vi "SMO Activity Tree.vi"   [LabVIEW 2021, in "smo.lvlib" / "SMO.lvclass"]
uses:
  SMO.lvclass
  SMO.lvclass/SMO.ctl
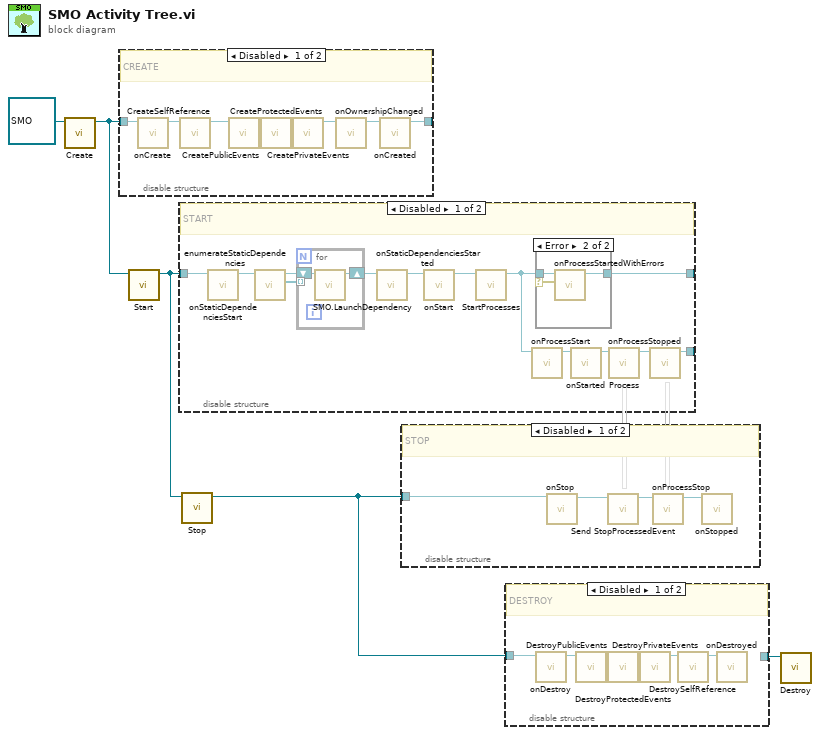
[diagram p0: block diagram]
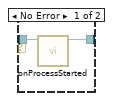
[diagram p4: hidden frame]
diagram:
  n1 = call "Create.vi"("SMO"=refnum<class "SMO.lvclass"> refnum) -> ("SMO out"=w3:refnum<class "SMO.lvclass">)  [unwired: 8 in, 2 out]
  n2 = disable-structure shown="Disabled" {
    disable-tunnel: w3 -> [w13 _]
    disable-tunnel: [w6 _] -> _
    frame Disabled {
      # "CREATE"
      n3 = call-dynamic "onCreate.vi"("SMO"=w13) -> ("SMO out"=w12:refnum<class "SMO.lvclass">)  [unwired: 9 in, 1 out]
      n4 = call-dynamic "CreateSelfReference.vi"("SMO"=w12) -> ("SMO out"=w11:refnum<class "SMO.lvclass">)  [unwired: 9 in, 1 out]
      n5 = call-dynamic "CreatePublicEvents.vi"("SMO"=w11) -> ("SMO out"=w10:refnum<class "SMO.lvclass">)  [unwired: 9 in, 1 out]
      n6 = call-dynamic "CreateProtectedEvents.vi"("SMO"=w10) -> ("SMO out"=w9:refnum<class "SMO.lvclass">)  [unwired: 9 in, 1 out]
      n7 = call-dynamic "CreatePrivateEvents.vi"("SMO"=w9) -> ("SMO out"=w8:refnum<class "SMO.lvclass">)  [unwired: 9 in, 1 out]
      n8 = call-dynamic "onOwnershipChanged.vi"("SMO in"=w8) -> ("SMO out"=w7:refnum<class "SMO.lvclass">)  [unwired: 9 in, 1 out]
      n9 = call-dynamic "onCreated.vi"("SMO"=w7) -> ("SMO out"=w6:refnum<class "SMO.lvclass">)  [unwired: 9 in, 1 out]
    }
    frame Enabled {
    }
  }
  n10 = call "Start.vi"("SMO"=w3) -> ("SMO out"=w4:refnum<class "SMO.lvclass">)  [unwired: 9 in, 1 out]
  n11 = disable-structure shown="Disabled" {
    disable-tunnel: w4 -> [w26 _]
    disable-tunnel: [w18 _] -> _
    disable-tunnel: [w17 _] -> _
    frame Disabled {
      # "START"
      n12 = call-dynamic "onStaticDependenciesStart.vi"("SMO"=w26) -> ("SMO out"=w24:refnum<class "SMO.lvclass">)  [unwired: 9 in, 1 out]
      n13 = call-dynamic "enumerateStaticDependencies.vi"("SMO"=w24) -> ("Static Dependencies"=w22:refnum<class "Dependency.lvclass">[], "SMO out"=w23:refnum<class "SMO.lvclass">)  [unwired: 8 in, 1 out]
      n14 = for {
        shift-right: [w33] -> w25
        shift-left: w23 -> [w32]
        tunnel: w22 -> [_] mode=indexing
        n15 = call "SMO.LaunchDependency.vi"("SMO in"=w32) -> ("SMO out"=w33:refnum<class "SMO.lvclass">)  [unwired: 7 in, 3 out]
      }
      n16 = call-dynamic "onStaticDependenciesStarted.vi"("SMO"=w25) -> ("SMO out"=w21:refnum<class "SMO.lvclass">)  [unwired: 9 in, 1 out]
      n17 = call-dynamic "onStart.vi"("SMO"=w21) -> ("SMO out"=w20:refnum<class "SMO.lvclass">)  [unwired: 9 in, 1 out]
      n18 = call "StartProcesses.vi"("SMO"=w20) -> ("SMO out"=w19:refnum<class "SMO.lvclass">)  [unwired: 9 in, 1 out]
      n19 = call-dynamic "onProcessStart.vi"("SMO"=w19) -> ("SMO out"=w16:refnum<class "SMO.lvclass">)  [unwired: 9 in, 1 out]
      n20 = case shown="Error" {
        selector: _ -> [_ w29]
        tunnel: w19 -> [w28 w31]
        tunnel: [w27 w30] -> w17
        frame No Error {
          n21 = call-dynamic "onProcessStarted.vi"("SMO"=w28) -> ("SMO out"=w27:refnum<class "SMO.lvclass">)  [unwired: 9 in, 1 out]
        }
        frame Error {
          n22 = call-dynamic "onProcessStartedWithErrors.vi"("Start error"=w29, "SMO"=w31) -> ("SMO out"=w30:refnum<class "SMO.lvclass">)  [unwired: 8 in, 1 out]
        }
      }
      n23 = call-dynamic "onStarted.vi"("SMO"=w16) -> ("SMO out"=w15:refnum<class "SMO.lvclass">)  [unwired: 9 in, 1 out]
      n24 = call-dynamic "Process.vi"("SMO"=w15) -> ("SMO out"=w14:refnum<class "SMO.lvclass">)  [unwired: 9 in, 1 out]
      n25 = call-dynamic "onProcessStopped.vi"("SMO"=w14) -> ("SMO out"=w18:refnum<class "SMO.lvclass">)  [unwired: 9 in, 1 out]
    }
    frame Enabled {
    }
  }
  n26 = call "Stop.vi"("SMO"=w4) -> ("SMO out"=w2:refnum<class "SMO.lvclass">)  [unwired: 9 in, 1 out]
  n27 = disable-structure shown="Disabled" {
    disable-tunnel: w2 -> [w37 _]
    frame Disabled {
      # "STOP"
      n28 = call-dynamic "onStop.vi"("SMO"=w37) -> ("SMO out"=w34:refnum<class "SMO.lvclass">)  [unwired: 9 in, 1 out]
      n29 = call "Send StopProcessedEvent.vi"("SMO"=w34) -> ("SMO out"=w35:refnum<class "SMO.lvclass">)  [unwired: 9 in, 1 out]
      n30 = call-dynamic "onProcessStop.vi"("SMO"=w35) -> ("SMO out"=w36:refnum<class "SMO.lvclass">)  [unwired: 9 in, 1 out]
      n31 = call-dynamic "onStopped.vi"("SMO"=w36) -> ()  [unwired: 9 in, 2 out]
    }
    frame Enabled {
    }
  }
  n32 = disable-structure shown="Disabled" {
    disable-tunnel: w2 -> [w43 w44]
    disable-tunnel: [_ w44] -> w1
    frame Disabled {
      # "DESTROY"
      n33 = call-dynamic "onDestroy.vi"("SMO"=w43) -> ("SMO out"=w42:refnum<class "SMO.lvclass">)  [unwired: 9 in, 1 out]
      n34 = call-dynamic "DestroyPublicEvents.vi"("SMO"=w42) -> ("SMO out"=w41:refnum<class "SMO.lvclass">)  [unwired: 9 in, 1 out]
      n35 = call-dynamic "DestroyProtectedEvents.vi"("SMO"=w41) -> ("SMO out"=w40:refnum<class "SMO.lvclass">)  [unwired: 9 in, 1 out]
      n36 = call-dynamic "DestroyPrivateEvents.vi"("SMO"=w40) -> ("SMO out"=w39:refnum<class "SMO.lvclass">)  [unwired: 9 in, 1 out]
      n37 = call-dynamic "DestroySelfReference.vi"("SMO"=w39) -> ("SMO out"=w38:refnum<class "SMO.lvclass">)  [unwired: 9 in, 1 out]
      n38 = call-dynamic "onDestroyed.vi"("SMO"=w38) -> ()  [unwired: 10 in, 1 out]
    }
    frame Enabled {
    }
  }
  n39 = call "Destroy.vi"("SMO"=w1) -> ()  [unwired: 10 in, 1 out]
